vi "功率算法.vi"(11 "内部参数":string) -> (2 "各种功率":string, 3 "功率dBm":dbl)   [LabVIEW 2015]
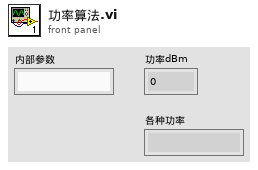
[diagram p1: front panel]
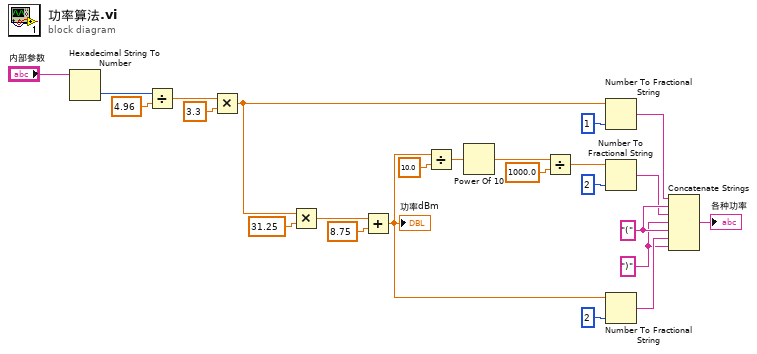
[diagram p0: block diagram]
diagram:
  w1 = ")" ("字符串")
  w3 = "(" ("字符串")
  n1 = Hexadecimal String To Number(string="内部参数") -> (number=w13:u32)  [unwired: 2 in, 1 out]
  n2 = Divide(x=w13, y=4.96) -> (x/y=w15:dbl)
  n3 = Multiply(x=w15, y=3.3) -> (x*y=w19:dbl)
  n4 = Multiply(x=w19, y=31.25) -> (x*y=w21:dbl)
  n5 = Add(x=w21, y=8.75) -> (x+y=w10:dbl)
  "功率dBm" <- w10
  n6 = Divide(x=w10, y=10.0) -> (x/y=w8:dbl)
  n7 = Power Of 10(x=w8) -> (10^x=w7:dbl)
  n8 = Divide(x=w7, y=1000.0) -> (x/y=w5:dbl)
  n9 = Number To Fractional String(number=w19, precision (6)=i16 1 ("精度(6)")) -> (F-format string=w17:string)  [unwired: 2 in]
  n10 = Number To Fractional String(number=w5, precision (6)=i16 2 ("精度(6)")) -> (F-format string=w2:string)  [unwired: 2 in]
  n11 = Number To Fractional String(number=w10, precision (6)=i16 2 ("精度(6)")) -> (F-format string=w24:string)  [unwired: 2 in]
  n12 = Concatenate Strings(w17, w3, w2, w1, w3, w24, w1) -> (→"各种功率":string)
